vi "Launcher.vi"() -> ()   [LabVIEW 2024]
panel:
  out "CableCount":dbl caption="Count"
  out "NutCount":dbl caption="Count"
  out "NailCount":dbl caption="Count"
  out "ScrewCount":dbl caption="Count"
  # "CABLE"
  # "NUT"
  # "NAIL"
  # "SCREW"
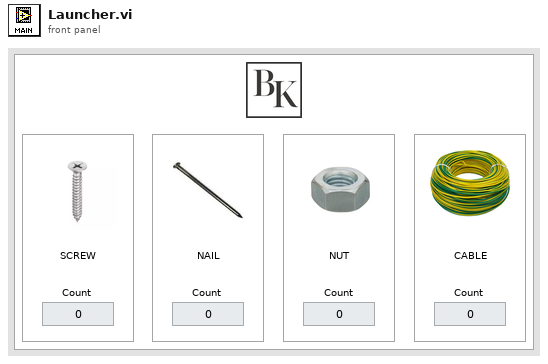
[diagram p1: front panel]
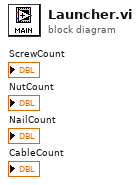
[diagram p0: block diagram]
diagram:
